vi "题目5.vi"() -> ()   [LabVIEW 2017]
panel:
  out "恭喜":bool
  out "通过":bool
  out "警告":bool
  in  "数值":dbl
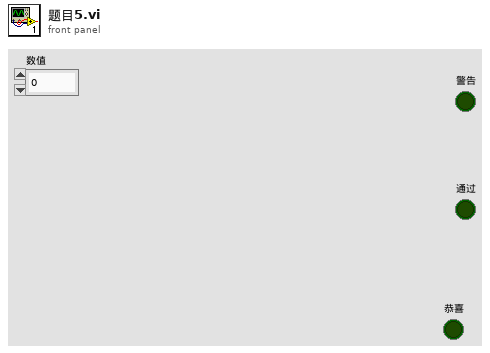
[diagram p1: front panel]
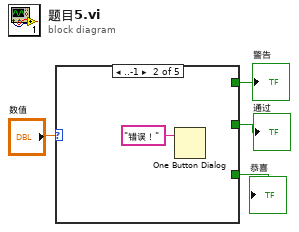
[diagram p0: block diagram]
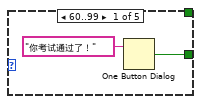
[diagram p2: hidden frame]
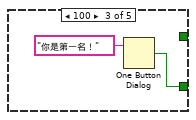
[diagram p3: hidden frame]
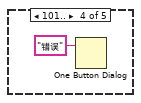
[diagram p4: hidden frame]
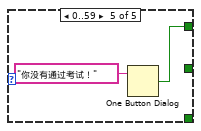
[diagram p5: hidden frame]
diagram:
  n1 = case shown="..-1" "数值" {
    tunnel: [_ _ _ _ w11] -> w2
    tunnel: [w5 _ _ _ _] -> w1
    tunnel: [_ _ w8 _ _] -> w3
    frame 60..99 {
      n2 = One Button Dialog(message="你考试通过了！" ("消息")) -> (true=w5:bool)  [unwired: 1 in]
    }
    frame ..-1 {
      n3 = One Button Dialog(message="错误！" ("消息")) -> ()  [unwired: 1 in, 1 out]
    }
    frame 100 {
      n4 = One Button Dialog(message="你是第一名！" ("消息")) -> (true=w8:bool)  [unwired: 1 in]
    }
    frame 101.. {
      n5 = One Button Dialog(message="错误" ("消息")) -> ()  [unwired: 1 in, 1 out]
    }
    frame 0..59 {
      n6 = One Button Dialog(message="你没有通过考试！" ("消息")) -> (true=w11:bool)  [unwired: 1 in]
    }
  }
  "警告" <- w2
  "通过" <- w1
  "恭喜" <- w3
